vi "Get_CODE_ID.vi"(11 "CODE_MAIN":string) -> (3 "CODE_ID":string)   [LabVIEW 2020]
uses:
  Global1.vi
panel:
  out "error out":errorcluster
  in  "error in (no error)":errorcluster
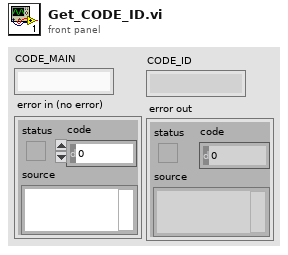
[diagram p1: front panel]
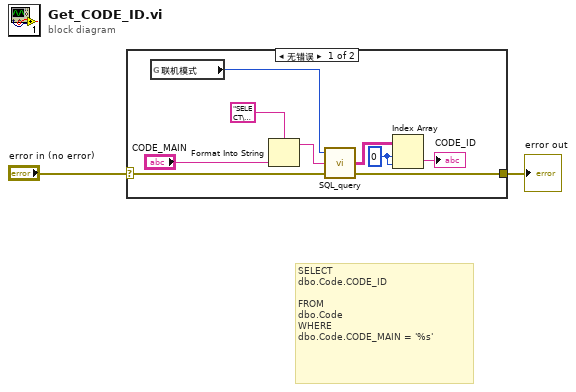
[diagram p0: block diagram]
diagram:
  # "SELECT\ndbo.Code.CODE_ID\n\nFROM\ndbo.Code\nWHERE\ndbo.Code.CODE_MAIN = '%s'"
  n1 = case shown="无错误" "error in (no error)" {
    selector: "error in (no error)" -> [w8 w12]
    tunnel: [w7 w12] -> w1
    frame No Error {
      w5 = 0 ("索引 (行)")
      n2 = global read "Global1.vi" "联机模式"() -> (w3:enum16{"单机", "追溯"})
      n3 = Format Into String(format string="SELECT\ndbo.Code.CODE_ID\n\nFROM\ndbo.Code\nWHERE\ndbo.Code.CODE_MAIN = '%s'" ("格式字符串"), "CODE_MAIN") -> (resulting string=w9:string)  [unwired: 2 in, 1 out]
      n4 = call "SQL_query.vi"("error in (no error)"=w8, "SQL query"=w9, "联机模式"=w3) -> ("error out"=w7:errorcluster, "data"=w6:string[][])  [unwired: 1 out]
      n5 = Index Array(array=w6, index (row)=w5, index (col)=w5) -> (element=→"CODE_ID":string)
    }
    frame Error {
    }
  }
  "error out" <- w1
